vi "_TEST_ObjCacher3.vi"() -> ()   [LabVIEW 2017]
uses:
  4d0ec281-761c-453f-b043-f57a17d307e5.vi
  93644015-ec6d-4267-aa01-dff2673081ed.vi
  f202f320-99f5-41a6-9dd7-7698db9a53b3.vi
  2509fc1b-10c8-4ef8-b539-dde5e3d1025b.vi
  ea14dd0e-9980-46cb-b21f-42c606d5dbd9.vi
  3aa4f933-e729-4c0d-be0d-f806621a85f5.vi
  b4b4f43b-d35a-4920-9647-6c5f1a3dc421.vi
  753ec2aa-3a5b-4aef-8294-15577f7a7708.vi
  3ef58916-56f3-49aa-81c9-1b75896433af.vi
  1468781d-bff3-4912-8551-fa98e2c574ff.vi
  742b683d-6189-41e9-b2a2-ecc88533b8bd.vi
  2f435e4a-757e-4ba5-9ca9-abbe54f1b102.vi
  10f2d8f1-de70-4874-a558-64f6e11ec28e.vi
  4a84e6f4-0222-429e-b57f-9413c1a2a4b9.vi
  2fba8e31-606a-475f-917b-8143bbd4d363.vi
  024cdb13-be77-41d8-b701-53d233da8922.vi
  d8522955-cbb2-42ea-80a8-12da07169ad9.vi
  403843ad-9117-42bc-9984-432dc07af900.vi
  93644015-ec6d-4267-aa01-dff2673081ed.vi/df97a732-2aa1-48ca-a021-ea6fe392e42b.vi
  f202f320-99f5-41a6-9dd7-7698db9a53b3.vi/e699d232-c896-4670-a9c5-e7dd2195749c.vi
  2509fc1b-10c8-4ef8-b539-dde5e3d1025b.vi/ccdad7bb-004e-4762-afb1-65ca7d6130ea.vi
  ea14dd0e-9980-46cb-b21f-42c606d5dbd9.vi/aaef58af-3a80-4898-9b69-f04cd84d0e55.vi
  3aa4f933-e729-4c0d-be0d-f806621a85f5.vi/aaef58af-3a80-4898-9b69-f04cd84d0e55.vi
  b4b4f43b-d35a-4920-9647-6c5f1a3dc421.vi/e699d232-c896-4670-a9c5-e7dd2195749c.vi
  753ec2aa-3a5b-4aef-8294-15577f7a7708.vi/aaef58af-3a80-4898-9b69-f04cd84d0e55.vi
  1468781d-bff3-4912-8551-fa98e2c574ff.vi/df97a732-2aa1-48ca-a021-ea6fe392e42b.vi
  742b683d-6189-41e9-b2a2-ecc88533b8bd.vi/e699d232-c896-4670-a9c5-e7dd2195749c.vi
  2f435e4a-757e-4ba5-9ca9-abbe54f1b102.vi/ccdad7bb-004e-4762-afb1-65ca7d6130ea.vi
  10f2d8f1-de70-4874-a558-64f6e11ec28e.vi/aaef58af-3a80-4898-9b69-f04cd84d0e55.vi
  4a84e6f4-0222-429e-b57f-9413c1a2a4b9.vi/aaef58af-3a80-4898-9b69-f04cd84d0e55.vi
  2fba8e31-606a-475f-917b-8143bbd4d363.vi/e699d232-c896-4670-a9c5-e7dd2195749c.vi
  024cdb13-be77-41d8-b701-53d233da8922.vi/aaef58af-3a80-4898-9b69-f04cd84d0e55.vi
  <userlib>/NEVSTOP-Programming-Palette/Application/Valid VI Reference_nevstop.vi
  d8522955-cbb2-42ea-80a8-12da07169ad9.vi/b7be58e1-3d0a-4835-8841-f13dfc0f9efe.vi
  d8522955-cbb2-42ea-80a8-12da07169ad9.vi/69f77548-5889-44c6-8640-e9f058736a5d.vi
  d8522955-cbb2-42ea-80a8-12da07169ad9.vi/ea8d3cea-2f8d-4420-9a60-a5294947b6ae.vi
  403843ad-9117-42bc-9984-432dc07af900.vi/69f77548-5889-44c6-8640-e9f058736a5d.vi
  403843ad-9117-42bc-9984-432dc07af900.vi/ea8d3cea-2f8d-4420-9a60-a5294947b6ae.vi
  403843ad-9117-42bc-9984-432dc07af900.vi/f4546358-8284-4e82-84b2-162a8f6e8dde.vi
  d8522955-cbb2-42ea-80a8-12da07169ad9.vi/b7be58e1-3d0a-4835-8841-f13dfc0f9efe.vi/ccdad7bb-004e-4762-afb1-65ca7d6130ea.vi
  403843ad-9117-42bc-9984-432dc07af900.vi/f4546358-8284-4e82-84b2-162a8f6e8dde.vi/aaef58af-3a80-4898-9b69-f04cd84d0e55.vi
  Data/_support/Get DataType Description String.vi
  _support/Resource.vi
  ObjectCacherAPI.lvlib
panel:
  out "String 2":string
  out "String":string
  out "names":string[](array[string])
  out "cacher 2":variant
  out "cacher":variant
  out "Global Cacher":variant
  out "error out":errorcluster
  out "Array 3":variant[](array[variant])
  out "Array 2":T1(array[cluster])
  out "Array":variant[](array[variant])
  out "Array 2":T1(array[cluster])
  out "Array 2":T1(array[cluster])
  out "Variant 2":T2
  out "Array":variant[](array[variant])
  out "Variant":string[](array[string])
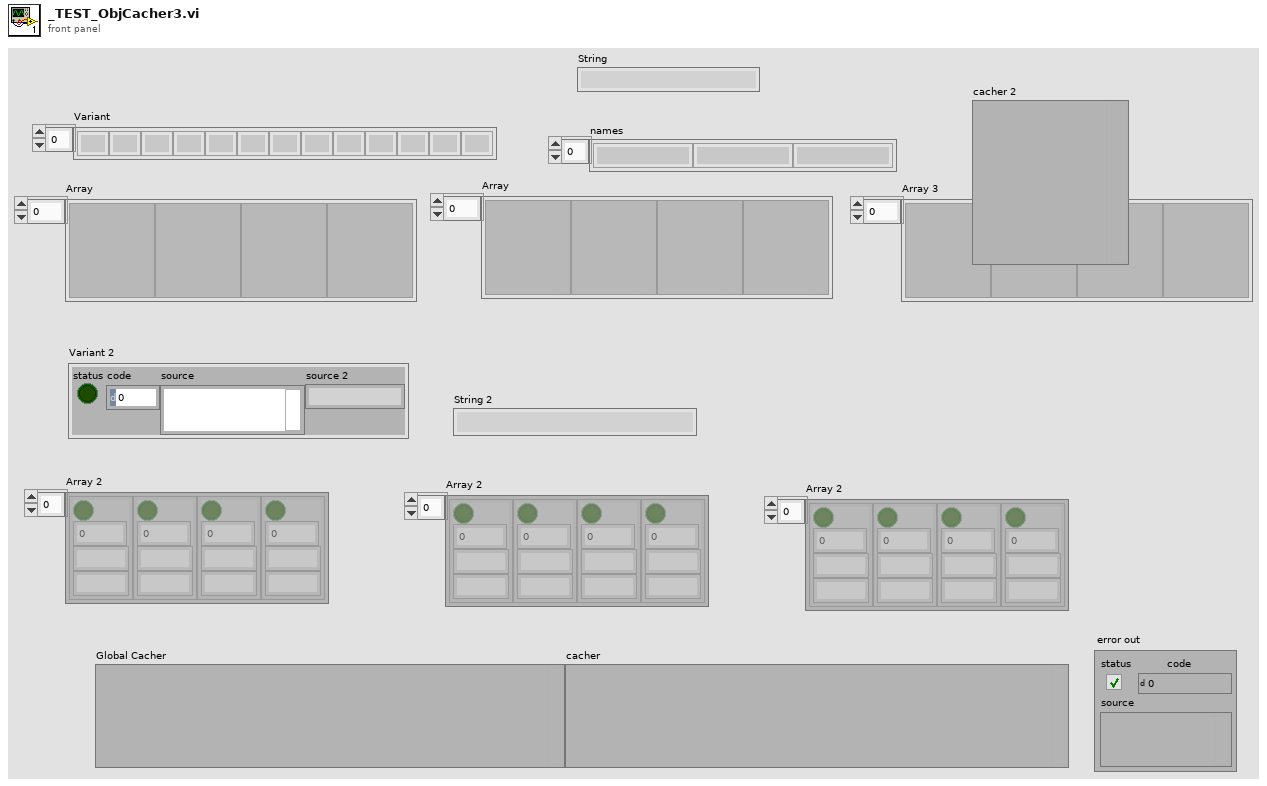
[diagram p1: front panel]
types:
  T1 = cluster{"status":bool, "code":i32, "source":string, "source 2":string}[]
  T2 = cluster{"status":bool, "code":i32, "source":string, "source 2":string}
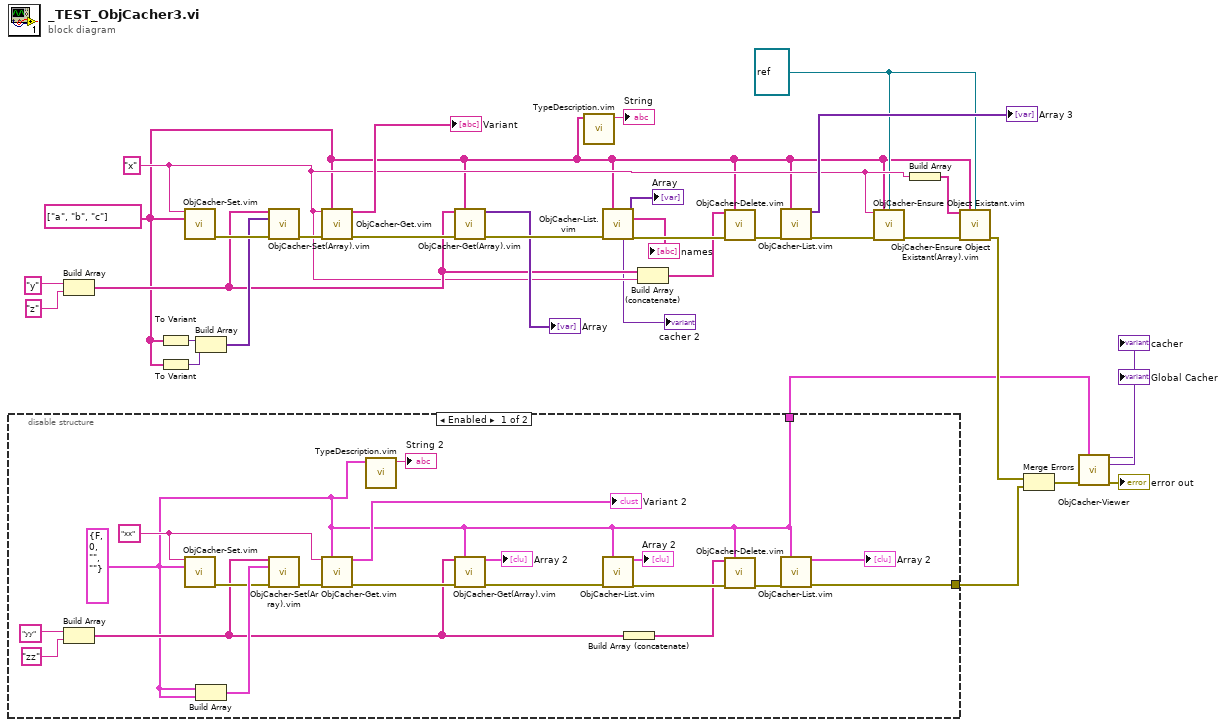
[diagram p0: block diagram]
diagram:
  w12 = refnum<vi> refnum ("Generator VI Ref")
  w14 = "x" ("Module Name")
  w3 = string[] ["a", "b", "c"]
  n1 = disable-structure shown="Enabled" {
    disable-tunnel: [w36 _] -> w9
    disable-tunnel: [w34 _] -> w1
    frame Enabled {
      w37 = "xx" ("Module Name")
      w34 = T2 {"status"=FALSE, "code"=0, "source"="", "source 2"=""}
      n2 = Build Array("yy" ("Module Name"), "zz" ("Module Name")) -> (w39:string[])
      n3 = call "ObjCacher-Set.vim"("Module Name"=w37, "data"=w34) -> ("error out"=w46:errorcluster)  [unwired: 11 in, 2 out]
      n4 = Build Array(w34, w34) -> (w49:T1)
      n5 = call "ObjCacher-Set(Array).vim"("Module Name"=w39, "data"=w49, "error in (no error)"=w46) -> ("error out"=w50:errorcluster)  [unwired: 10 in, 2 out]
      n6 = call "ObjCacher-Get.vim"("Module Name"=w37, "type"=w34, "error in (no error)"=w50) -> ("Variant"=→"Variant 2":T2, "error out"=w51:errorcluster)  [unwired: 9 in, 2 out]
      n7 = call "TypeDescription.vim"("type"=w34) -> ("String"=→"String 2":string)  [unwired: 9 in, 1 out]
      n8 = call "ObjCacher-Get(Array).vim"("Module Name"=w39, "type"=w34, "error in (no error)"=w51) -> ("Array"=→"Array 2":T1, "error out"=w52:errorcluster)  [unwired: 9 in, 2 out]
      n9 = call "ObjCacher-List.vim"("Variant"=w34, "error in (no error)"=w52) -> ("Array"=→"Array 2":T1, "error out"=w42:errorcluster)  [unwired: 10 in, 2 out]
      n10 = Build Array (concatenate)(w39) -> (w38:string[])
      n11 = call "ObjCacher-Delete.vim"("Module Name"=w38, "type"=w34, "error in (no error)"=w42) -> ("error out"=w41:errorcluster)  [unwired: 10 in, 2 out]
      n12 = call "ObjCacher-List.vim"("Variant"=w34, "error in (no error)"=w41) -> ("Array"=→"Array 2":T1, "error out"=w36:errorcluster)  [unwired: 10 in, 2 out]
    }
    frame Disabled {
    }
  }
  n13 = Build Array("y" ("Module Name"), "z" ("Module Name")) -> (w17:string[])
  n14 = To Variant(anything=w3) -> (Variant=w27:variant)
  n15 = To Variant(anything=w3) -> (Variant=w28:variant)
  n16 = call "ObjCacher-Set.vim"("Module Name"=w14, "data"=w3) -> ("error out"=w31:errorcluster)  [unwired: 11 in, 2 out]
  n17 = Build Array(w27, w28) -> (w26:variant[])
  n18 = call "ObjCacher-Set(Array).vim"("Module Name"=w17, "data"=w26, "error in (no error)"=w31) -> ("error out"=w25:errorcluster)  [unwired: 10 in, 2 out]
  n19 = call "ObjCacher-Get.vim"("Module Name"=w14, "type"=w3, "error in (no error)"=w25) -> ("Variant"=→"Variant":string[], "error out"=w24:errorcluster)  [unwired: 9 in, 2 out]
  n20 = call "ObjCacher-Get(Array).vim"("Module Name"=w17, "type"=w3, "error in (no error)"=w24) -> ("Array"=→"Array":variant[], "error out"=w23:errorcluster)  [unwired: 9 in, 2 out]
  n21 = call "TypeDescription.vim"("type"=w3) -> ("String"=→"String":string)  [unwired: 9 in, 1 out]
  n22 = call "ObjCacher-List.vim"("Variant"=w3, "error in (no error)"=w23) -> ("Array"=→"Array":variant[], "names"=→"names":string[], "cacher"=→"cacher 2":variant, "error out"=w20:errorcluster)  [unwired: 10 in]
  n23 = Build Array (concatenate)(w17, w14) -> (w18:string[])
  n24 = call "ObjCacher-Delete.vim"("Module Name"=w18, "type"=w3, "error in (no error)"=w20) -> ("error out"=w21:errorcluster)  [unwired: 10 in, 2 out]
  n25 = call "ObjCacher-List.vim"("Variant"=w3, "error in (no error)"=w21) -> ("Array"=→"Array 3":variant[], "error out"=w15:errorcluster)  [unwired: 10 in, 2 out]
  n26 = call "ObjCacher-Ensure Object Existant.vim"("Module Name"=w14, "type"=w3, "Generator VI Ref"=w12, "error in (no error)"=w15) -> ("error out"=w16:errorcluster)  [unwired: 8 in, 3 out]
  n27 = Build Array(w14) -> (w13:string[])
  n28 = call "ObjCacher-Ensure Object Existant(Array).vim"("Module Name"=w13, "type"=w3, "Generator VI Ref"=w12, "error in (no error)"=w16) -> ("error out"=w11:errorcluster)  [unwired: 9 in, 2 out]
  n29 = Merge Errors(w11, w9) -> (w10:errorcluster)
  n30 = call "ObjCacher-Viewer.vi"("type"=w1, "error in (no error)"=w10) -> ("cacher"=→"cacher":variant, "Global Cacher"=→"Global Cacher":variant, "error out"=→"error out":errorcluster)  [unwired: 11 in]
